vi "SL_Straight_Edge_Detection.vi"(8 "error in":errorcluster, 11 "Image In":T1) -> (0 "error out":errorcluster, 2 "Image":T1(plugin-control), 3 "Image Out":T1)   [LabVIEW 2015]
doc: "This example shows how to use Find Straight Edges in NI Vision. Find Straight Edges finds lines (or straight edges) within a search region. Find Straight Edges is a precursor function to many of the gauging and inspection tasks. For example, the location of the straight edges found within a region that encloses an object can interpreted as the boundaries of the object whose dimensions have to be measured for a gauging application or the presence of a crack in the surface of an object for an inspection application."
uses:
  <vilib>/vision/Image Controls.llb/IMAQ Image.ctl
  <vilib>/vision/NI_Vision_Development_Module.lvlib
panel:
  out "Number of Lines Found":i32
  in  "Line Options":T2={"Number of Lines"=6, "Type"=4, "Minimum Score"=100.0, "Maximum Score"=1024.0, "Orientation"=0.0, "Angle Range"=10.0, "Angle Tolerance"=1.0, "Step Size"=3, "Min. SNR (db)"=0.0, "Min. Points (%)"=25.0, "Hough Iterations"=5} {"Min. Points (%)" min=0.0 max=100.0; "Min. SNR (db)" min=0.0; "Maximum Score" min=0.0 max=1024.0; "Minimum Score" min=1.0 max=1024.0 step=1.0; "Type" items=["First Edge Rake", "Best Edge Rake", "Hough Edge Rake", "First Edge Projection", "Best Edge Projection"]}
  in  "Edge Options":T3={"Edge Polarity"=0, "Kernel Size"=5, "Width"=3, "Minimum Edge Strength"=50.0, "Interpolation Type"=1, "Data Processing Method"=0} {"Data Processing Method" items=["Average", "Median"]; "Interpolation Type" items=["Zero Order"=0, "Bilinear"=1, "Bilinear Fixed"=4]; "Minimum Edge Strength" min=0.0 max=255.0 format="%.2g"; "Width" min=1 step=2; "Kernel Size" min=3 step=2; "Edge Polarity" items=["All Edges", "Rising Edges", "Falling Edges"]}
  in  "Search Direction":u32(ring) items=["Left to Right", "Right to Left", "Top to Bottom", "Bottom to Top"]
  in  "Stop":bool
  # "Overview: Demonstrates how to use the IMAQ Find Straight Edges function to find multiple straight lines in the Region of Interest (ROI).\nRequirements: Vision Development Software.\nInstructions: \n1. Run the VI.\n2. Draw a Region of Interest in the image, or modify the Edge Options or Line Options to see the straight edges the algorithm detects."
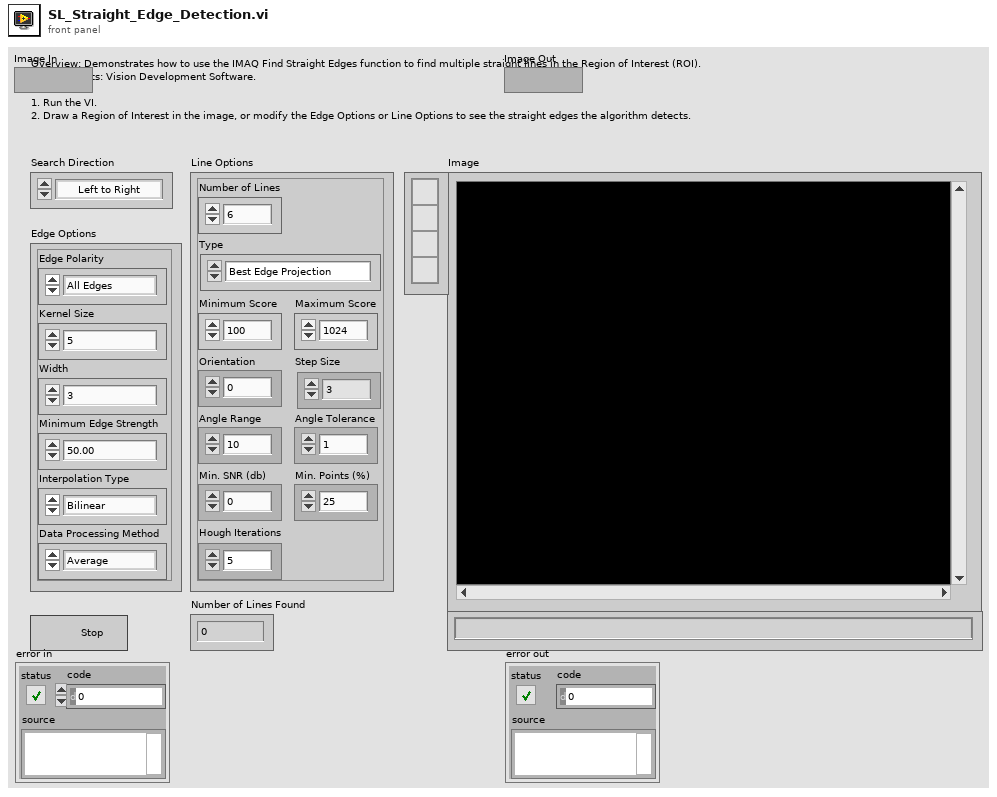
[diagram p1: front panel]
types:
  T1 = typedef "IMAQ Image.ctl" = refnum<image>
  T2 = cluster{"Number of Lines":i32, "Type":u16, "Minimum Score":dbl, "Maximum Score":dbl, "Orientation":dbl, "Angle Range":dbl, "Angle Tolerance":dbl, "Step Size":u32, "Min. SNR (db)":dbl, "Min. Points (%)":dbl, "Hough Iterations":i32}
  T3 = cluster{"Edge Polarity":u16, "Kernel Size":u32, "Width":u32, "Minimum Edge Strength":dbl, "Interpolation Type":u16, "Data Processing Method":u16}
  T4 = typedef "IMAQ Rectangle" = cluster{"Left":i32, "Top":i32, "Right":i32, "Bottom":i32, "Rotation":dbl}
  T5 = typedef "ROI Descriptor" = cluster{"Global Rectangle":i32[], "Contours":cluster{"ID":enum32{"External", "Internal"}, "Type":u32, "Coordinates":i32[]}[]}
  T6 = cluster{"Global Rectangle":i32[], "Contours":cluster{"Contour Type":u32, "ROI Type":u32, "Points":i32[]}[]}
  T7 = cluster{"Point1 (Pixels)":cluster{"X":sgl, "Y":sgl}, "Point2 (Pixels)":cluster{"X":sgl, "Y":sgl}, "Point1 (Real-World)":cluster{"X":sgl, "Y":sgl}, "Point2 (Real-World)":cluster{"X":sgl, "Y":sgl}, "Angle (Pixel)":dbl, "Angle (Real-World)":dbl, "Score":dbl, "Straightness":dbl, "Average SNR (db)":dbl, "Calibration Valid":bool}[]
  T8 = typedef "Search Line.ctl" = cluster{"Start Point":cluster{"X":sgl, "Y":sgl}, "End Point":cluster{"X":sgl, "Y":sgl}, "Edge Info":T9[], "Edge Map":dbl[], "Calibration Valid":bool}
  T9 = typedef "Edge New.ctl" = cluster{"Location (Pixel)":cluster{"X":sgl, "Y":sgl}, "Location (Real-World)":cluster{"X":sgl, "Y":sgl}, "Distance (Pixel)":dbl, "Distance (Real-World)":dbl, "Strength":dbl, "Noise":dbl, "Rising?":bool}
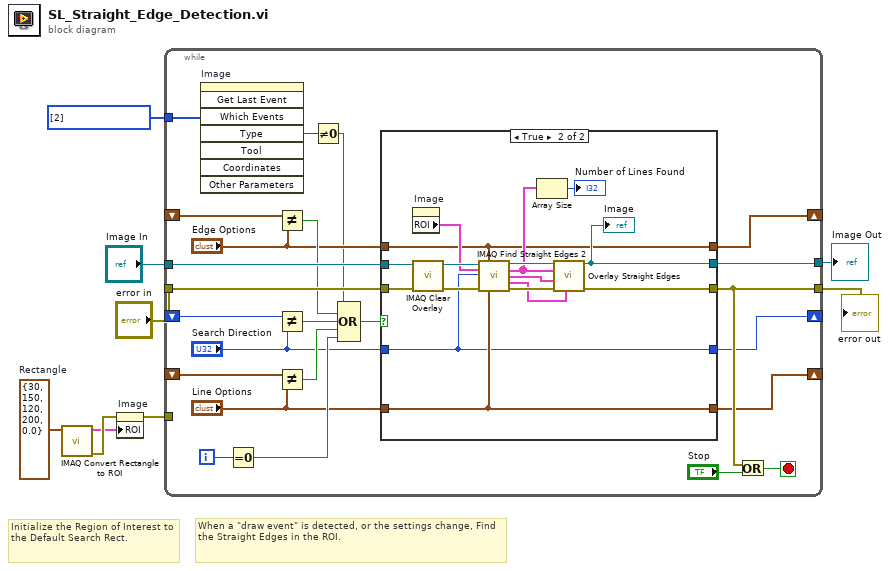
[diagram p0: block diagram]
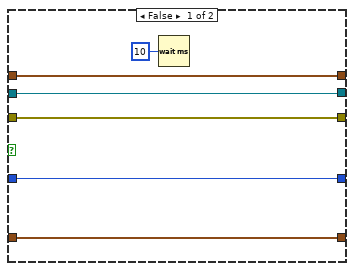
[diagram p2: hidden frame]
diagram:
  w8 = i32[] [2] items=["No Event"=0, "Click Event"=1, "Draw Event"=2, "Size Event"=4, "Scroll Event"=5, "Double Click Event"=8] ("Which Events")
  w9 = T4 {"Left"=30, "Top"=150, "Right"=120, "Bottom"=200, "Rotation"=0.0}  # Rectangle
  # "When a \"draw event\" is detected, or the settings change, Find the Straight Edges in the ROI."
  # "Initialize the Region of Interest to the Default Search Rect."
  n1 = call "IMAQ Convert Rectangle to ROI"("Rectangle"=w9) -> ("error out"=w7:errorcluster, "ROI Descriptor"=w6:T5)  [unwired: 8 in]
  n2 = property on="Image" class="ImageControl"(error in=w7, "ROI"=w6) -> (error out=w5:errorcluster)  [unwired: 1 in, 1 out]
  n3 = while {
    tunnel: "Image In" -> [w33]
    tunnel: [w17] -> w1
    tunnel: [w32] -> w2
    tunnel: "error in" -> [w31]
    shift-right: [w10] -> _
    shift-left: _ -> [w28]
    shift-right: [w11] -> _
    shift-left: _ -> [w30]
    shift-right: [w12] -> _
    shift-left: _ -> [w29]
    tunnel: w8 -> [w15]
    tunnel: w5 -> [_]
    i -> [w27]
    stop <- w16 stop-if-true
    n4 = invoke on="Image" class="ImageControl" method="Get Last Event"("Which Events"=w15) -> ("Type"=w14:i32)  [unwired: 7 in, 7 out]
    n5 = Equal To 0?(x=w27) -> (x = 0?=w23:bool)
    n6 = Not Equal?(x=w28, y="Edge Options") -> (x != y?=w22:bool)
    n7 = Not Equal?(x=w30, y="Search Direction") -> (x != y?=w26:bool)
    n8 = Not Equal?(x=w29, y="Line Options") -> (x != y?=w24:bool)
    n9 = Not Equal To 0?(x=w14) -> (x != 0?=w13:bool)
    n10 = Compound Arithmetic op=OR(w13, w22, w26, w24, w23) -> (w25:bool)
    n11 = case shown="True" w25 {
      tunnel: w33 -> [w39 w55]
      tunnel: [w39 w54] -> w32
      tunnel: w31 -> [w38 w53]
      tunnel: [w38 w52] -> w17
      tunnel: "Edge Options" -> [w34 w40]
      tunnel: "Search Direction" -> [w36 w41]
      tunnel: "Line Options" -> [w37 w42]
      tunnel: [w37 w42] -> w12
      tunnel: [w36 w41] -> w11
      tunnel: [w34 w40] -> w10
      frame False {
        n12 = Wait (ms)(milliseconds to wait=u32 10) -> ()  [unwired: 1 out]
      }
      frame True {
        n13 = property on="Image" class="ImageControl"() -> ("ROI"=w49:T6)  [unwired: 2 in, 2 out]
        n14 = call "IMAQ Clear Overlay"("error in (no error)"=w53, "Image"=w55) -> ("error out"=w51:errorcluster, "Image Out"=w50:T1)  [unwired: 8 in]
        n15 = call "IMAQ Find Straight Edges 2"("Image"=w50, "Edge Options"=w40, "ROI Descriptor"=w49, "Search Direction"=w41, "error in (no error)"=w51, "Line Options"=w42) -> ("Image (duplicate)"=w48:T1, "Straight Edges"=w44:T7, "Search Lines Information"=w47:T8[], "Used Edges"=w45:cluster{"Edge Information":T9[]}[], "error out"=w46:errorcluster)  [unwired: 5 in]
        n16 = Array Size(array=w44) -> (size(s)=→"Number of Lines Found":i32)
        n17 = call "Overlay Straight Edges.vi"("All Edges (Pixel)"=w45, "error in"=w46, "Search Lines Information"=w47, "Straight Edges"=w44, "Image In"=w48) -> ("error out"=w52:errorcluster, "Image Out"=w54:T1)  [unwired: 5 in]
        "Image" <- w54
      }
    }
    n18 = Or(x=w17, y="Stop") -> (x .or. y?=w16:bool)
  }
  "Image Out" <- w2
  "error out" <- w1
